vi "Store Static VI References for Subpanel.vi"(8 "error in (no error)":errorcluster, 11 "monitor configuration in":refnum<class "CCD monitor configuration.lvclass">) -> (0 "error out":errorcluster, 3 "monitor configuration out":refnum<class "CCD monitor configuration.lvclass">)   [LabVIEW 2016, in "CCD monitor.lvlib" / "CCD monitor configuration.lvclass"]
uses:
  <userlib>/Common Components/Hardware/Abstract System/Monitor/CCD monitor configuration.lvclass
  C:/Program Files (x86)/National Instruments/LabVIEW 2016/user.lib/Configuration Dialog Actor/Configuration.lvclass
  <userlib>/Configuration Dialog Actor/Configuration.lvclass
  <userlib>/Common Components/Hardware/CCD/CCD Configuration.lvclass
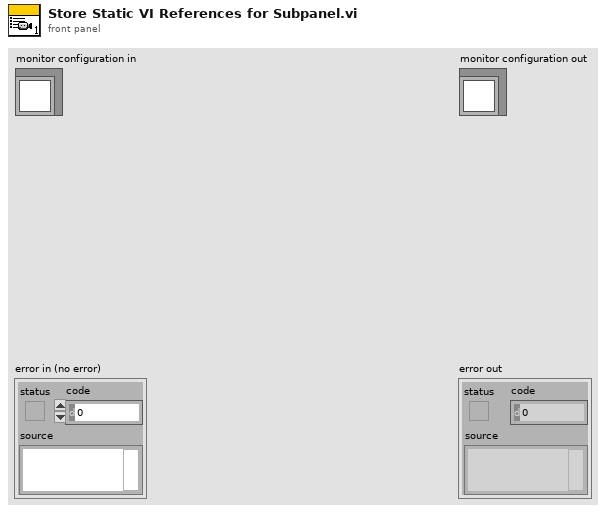
[diagram p1: front panel]
types:
  T1 = typedef "Configuration.lvlib/Configuration.lvclass/Data Retrieved by Lookup Table.ctl" = cluster{"VI Refnum":refnum<vi>, "Help Text":string}
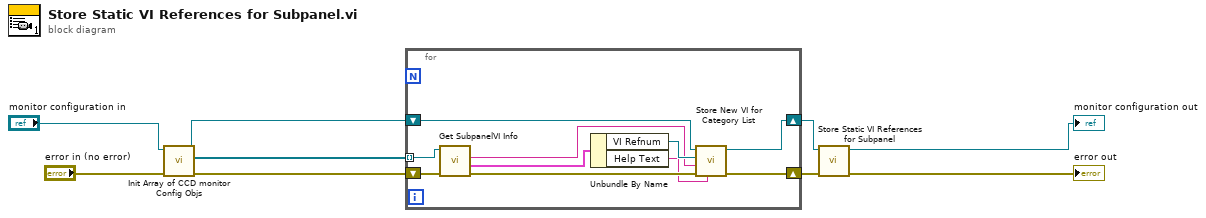
[diagram p0: block diagram]
diagram:
  n1 = call <userlib>:"Init Array of CCD monitor Config Objs.vi"("error in (no error)"="error in (no error)", "Hardware.lvlib:CCD monitor.lvlib:CCD monitor configuration.lvclass"="monitor configuration in") -> ("error out"=w4:errorcluster, "Array of CCD monitor"=w6:refnum<class "CCD Configuration.lvclass">[], "reference out"=w3:refnum<class "CCD monitor configuration.lvclass">)  [unwired: 7 in]
  n2 = for {
    tunnel: w6 -> [w19] mode=indexing
    shift-right: [w14] -> w1
    shift-left: w4 -> [w18]
    shift-right: [w10] -> w2
    shift-left: w3 -> [w11]
    n3 = call <userlib>:"Get SubpanelVI Info.vi"("error in (no error)"=w18, "Hardware.lvlib:CCD.lvlib:CCD Configuration.lvclass"=w19) -> ("error out"=w15:errorcluster, "Subpanel VI data"=w17:T1, "Category string"=w12:string)  [unwired: 6 in, 1 out]
    n4 = Unbundle By Name(w17) -> ("VI Refnum"=w16:refnum<vi>, "Help Text"=w13:string)
    n5 = call <userlib>:"Store New VI for Category List.vi"("Help Text"=w13, "error in (no error)"=w15, "String"=w12, "VI Refnum"=w16, "Configuration in"=w11) -> ("error out"=w14:errorcluster, "Configuration out"=w10:refnum<class "CCD monitor configuration.lvclass">)  [unwired: 5 in]
  }
  n6 = call-parent "Store Static VI References for Subpanel.vi"("error in (no error)"=w1, "Configuration in"=w2) -> ("error out"=→"error out":errorcluster, "Configuration out"=→"monitor configuration out":refnum<class "CCD monitor configuration.lvclass">)  [unwired: 8 in]
